vi "cycleAllNLMethods_invP.vi"() -> ()   [LabVIEW 2014] (continued)
  T3 = cluster{"invParams":cluster{"nlParams":T1, "qp0":dbl[], "q0dn":dbl[], "q0up":dbl[], "kn0":cluster{"tx01":dbl, "ty01":dbl, "tz01":dbl, "ry01":dbl, "rz01":dbl, "tx23":dbl, "ry34":dbl, "rz34":dbl, "cathL":dbl, "ry45":dbl, "rz45":dbl}, "knPM":cluster{"tx01":dbl, "ty01":dbl, "tz01":dbl, "ry01":dbl, "rz01":dbl, "tx23":dbl, "ry34":dbl, "rz34":dbl, "cathL":dbl, "ry45":dbl, "rz45":dbl}}, "qps0out":dbl[], "kn":T2, "fmin":dbl, "retCodeOut":i32}[]
  T4 = typedef "NI_Matrix.lvlib/RealMatrix.ctl" = dbl[][]
  T5 = cluster{"jointQps":dbl[], "ascH05":T4, "poseGRF":T4}[]
  T6 = typedef "homeBus.ctl" = cluster{"servo":cluster{"IP":string, "send to port":u16, "udpID":refnum<k16>}, "err":errorcluster, "jntLims":T7, "ts [ms]":dbl, "vLim":dbl[], "cmdQps":dbl[][], "asc":T8}
  T7 = typedef "jntLims.ctl" = cluster{"dn":dbl[], "up":dbl[]}
  T8 = typedef "ascSetup.ctl" = cluster{"resetOnInit":bool, "ang0":dbl[], "ang1":dbl[], "ang2":dbl[], "DataFormatType":i32}
  T9 = cluster{"invParams":cluster{"nlParams":T1, "qp0":dbl[], "q0dn":dbl[], "q0up":dbl[], "kn0":cluster{"tx01":dbl, "ty01":dbl, "tz01":dbl, "ry01":dbl, "rz01":dbl, "tx23":dbl, "ry34":dbl, "rz34":dbl, "cathL":dbl, "ry45":dbl, "rz45":dbl}, "knPM":cluster{"tx01":dbl, "ty01":dbl, "tz01":dbl, "ry01":dbl, "rz01":dbl, "tx23":dbl, "ry34":dbl, "rz34":dbl, "cathL":dbl, "ry45":dbl, "rz45":dbl}}, "qpStart":dbl[], "qpEnd":dbl[], "homeBus":T6}
  T10 = enum16{"GN_DIRECT", "GN_DIRECT_L", "GN_DIRECT_L_NOSCAL", "GN_DIRECT_L_RAND", "GN_DIRECT_L_RAND_NOSCAL", "GN_DIRECT_NOSCAL", "GN_ESCH", "GN_ISRES", "GN_MLSL", "GN_MLSL_LDS", "GN_ORIG_DIRECT", "GN_ORIG_DIRECT_L", "LN_BOBYQA", "LN_COBYLA", "LN_NELDERMEAD", "LN_NEWUOA", "LN_NEWUOA_BOUND", "LN_PRAXIS", "LN_SBPLX"}[]
  T11 = cluster{"nlParams":T1, "qp0":dbl[], "q0dn":dbl[], "q0up":dbl[], "kn0":cluster{"tx01":dbl, "ty01":dbl, "tz01":dbl, "ry01":dbl, "rz01":dbl, "tx23":dbl, "ry34":dbl, "rz34":dbl, "cathL":dbl, "ry45":dbl, "rz45":dbl}, "knPM":cluster{"tx01":dbl, "ty01":dbl, "tz01":dbl, "ry01":dbl, "rz01":dbl, "tx23":dbl, "ry34":dbl, "rz34":dbl, "cathL":dbl, "ry45":dbl, "rz45":dbl}}
  T12 = cluster{"invParams":cluster{"nlParams":T1, "qp0":dbl[], "q0dn":dbl[], "q0up":dbl[], "kn0":cluster{"tx01":dbl, "ty01":dbl, "tz01":dbl, "ry01":dbl, "rz01":dbl, "tx23":dbl, "ry34":dbl, "rz34":dbl, "cathL":dbl, "ry45":dbl, "rz45":dbl}, "knPM":cluster{"tx01":dbl, "ty01":dbl, "tz01":dbl, "ry01":dbl, "rz01":dbl, "tx23":dbl, "ry34":dbl, "rz34":dbl, "cathL":dbl, "ry45":dbl, "rz45":dbl}}, "qps0out":dbl[], "kn":T2, "fmin":dbl, "retCodeOut":i32}
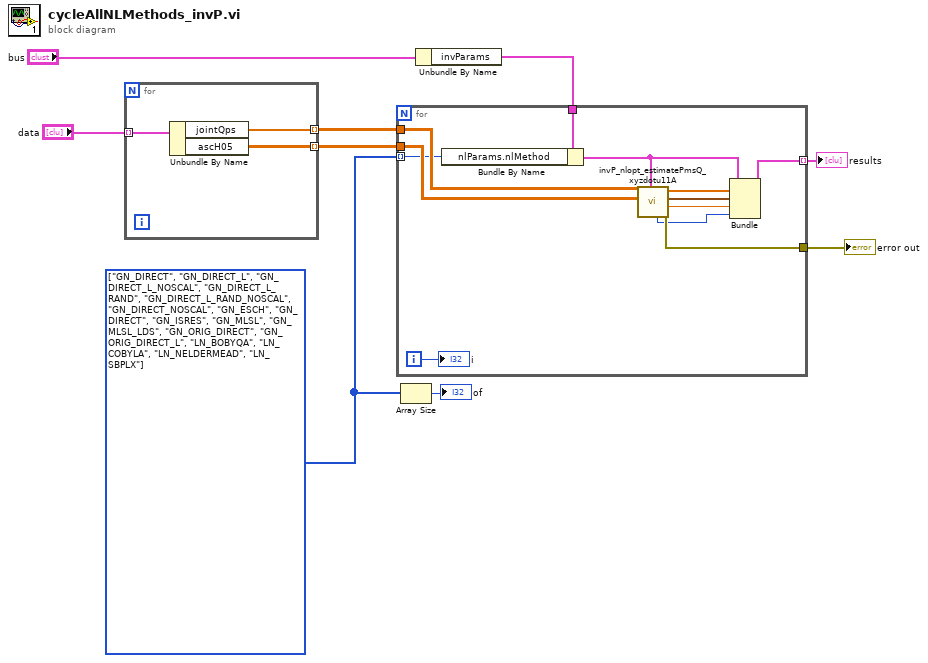
[diagram p0: block diagram]
diagram:
  w3 = T10 [enum."GN_DIRECT", enum."GN_DIRECT_L", enum."GN_DIRECT_L_NOSCAL", enum."GN_DIRECT_L_RAND", enum."GN_DIRECT_L_RAND_NOSCAL", enum."GN_DIRECT_NOSCAL", enum."GN_ESCH", enum."GN_DIRECT", enum."GN_ISRES", enum."GN_MLSL", enum."GN_MLSL_LDS", enum."GN_ORIG_DIRECT", enum."GN_ORIG_DIRECT_L", enum."LN_BOBYQA", enum."LN_COBYLA", enum."LN_NELDERMEAD", enum."LN_SBPLX"] items=["GN_DIRECT", "GN_DIRECT_L", "GN_DIRECT_L_NOSCAL", "GN_DIRECT_L_RAND", "GN_DIRECT_L_RAND_NOSCAL", "GN_DIRECT_NOSCAL", "GN_ESCH", "GN_ISRES", "GN_MLSL", "GN_MLSL_LDS", "GN_ORIG_DIRECT", "GN_ORIG_DIRECT_L", "LN_BOBYQA", "LN_COBYLA", "LN_NELDERMEAD", "LN_NEWUOA", "LN_NEWUOA_BOUND", "LN_PRAXIS", "LN_SBPLX"]
  n1 = for {
    tunnel: "data" -> [w12] mode=indexing
    tunnel: [w11] -> w9 mode=indexing
    tunnel: [w10] -> w8 mode=indexing
    n2 = Unbundle By Name(w12) -> ("jointQps"=w11:dbl[], "ascH05"=w10:T4)
  }
  n3 = Array Size(array=w3) -> (size(s)=→"of":i32)
  n4 = Unbundle By Name("bus") -> ("invParams"=w6:T11)
  n5 = for {
    tunnel: w9 -> [w24]
    tunnel: w8 -> [w22]
    tunnel: w6 -> [w20]
    tunnel: [w23] -> w4
    tunnel: w3 -> [w19] mode=indexing
    tunnel: [w13] -> w1 mode=indexing
    i -> [w21]
    n6 = Bundle By Name(cluster=w20, "nlParams.nlMethod"=w19) -> (w18:T11)
    n7 = call "invP_nlopt_estimatePmsQ_xyzdotu11A.vi"("in"=w18, "ascH05"=w22, "jointQps"=w24) -> ("error out"=w23:errorcluster, "fmin"=w15:dbl, "kn"=w16:T2, "qps0out"=w17:dbl[], "retCodeOut"=w14:i32)  [unwired: 4 in]
    n8 = Bundle("invParams"=w18, "qps0out"=w17, "kn"=w16, "fmin"=w15, "retCodeOut"=w14) -> (w13:T12)  [unwired: 1 in]
    "i" <- w21
  }
  "error out" <- w4
  "results" <- w1
